vi "NTJ_Build NT Field ID Buffer.vi"(11 "Field ID":i32) -> (3 "Data Buffer":string)   [LabVIEW 2019]
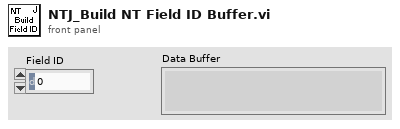
[diagram p1: front panel]
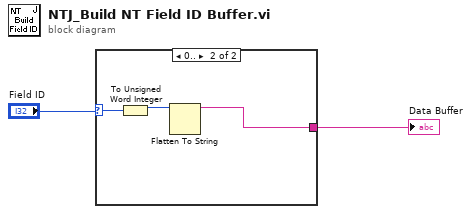
[diagram p0: block diagram]
diagram:
  n1 = case shown="0.." "Field ID" {
    selector: "Field ID" -> [_ w5]
    tunnel: [_ w3] -> w1
    frame Default {
    }
    frame 0.. {
      n2 = To Unsigned Word Integer(number=w5) -> (unsigned 16bit integer=w4:u16)
      n3 = Flatten To String(anything=w4) -> (data string=w3:string)  [unwired: 3 in, 2 out]
    }
  }
  "Data Buffer" <- w1
